vi "Bool2String.vi"(1 "布尔":bool) -> (0 "字符串":string)   [LabVIEW 2019]
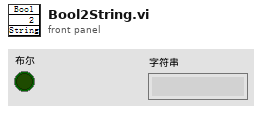
[diagram p1: front panel]
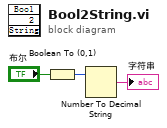
[diagram p0: block diagram]
diagram:
  n1 = Boolean To (0,1)(Boolean="布尔") -> (0, 1=w2:i16)
  n2 = Number To Decimal String(number=w2) -> (decimal integer string=→"字符串":string)  [unwired: 1 in]
